vi "Set Dev Format.vi"(8 "error in (no error)":errorcluster, 9 "firmware revision":string(combo), 10 "dev format":T1 {"loss format (0)" min=0 max=4; "cap format (0)" min=0 max=4}, 11 "VISA resource name":refnum<visa-resource-name>) -> (0 "error out":errorcluster, 2 "bridge error":T2, 3 "VISA resource name out":refnum<visa-resource-name>)   [LabVIEW 2024, in "Andeen-Hagerling 2700A.lvlib"]
doc: "Set the value of the deviation mode format parameter.\n\n0 - Deviation measurement results are\n reported in absolute pF and jpF units. A\n measurement at the Deviation Setpoint will\n be reported as DPointC pF and DPointL\n jpF.\n1 - Deviation measurement results are\n reported as simple differences from the\n Deviation Setpoint in units of pF and jpF.\n A measurement at the Deviation Setpoint\n will be reported as 0 pF and 0 jpF.\n2 Deviation measurement results are\n reported as differences from the Deviation\n Setpoint as a percentage of the Deviation\n Setpoint. A measurement at the Deviation\n Setpoint will be reported as 0% for both\n capacitance and loss.\n3 Deviation measurement results are\n reported as differences from the Deviation\n Setpoint as a percentage of the deviation\n input span. Measurement values at the\n DBndLo and DBndUp bounds will be\n reported as -50% and +50% respectively.\n4 Deviation measurement results are\n reported as differences from the Deviation\n Setpoint as a percentage of the deviation\n input span. Measurement values at the\n DBndLo and DBndUp bounds will be\n reported as -100% and +100% respectively."
uses:
  Andeen-Hagerling 2700A.lvlib
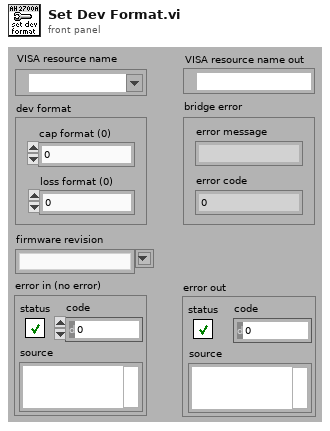
[diagram p1: front panel]
types:
  T1 = cluster{"cap format (0)":i32, "loss format (0)":i32}
  T2 = cluster{"error message":string, "error code":i32}
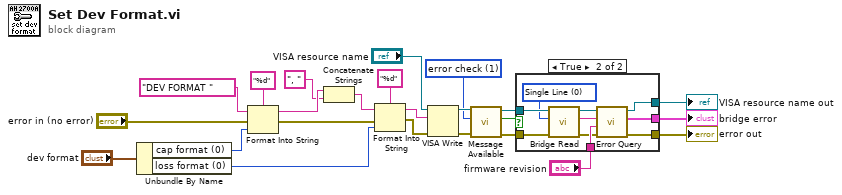
[diagram p0: block diagram]
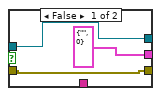
[diagram p2: hidden frame]
diagram:
  w1 = u16 1 items=["none", "error check", "multiline read", "infinite"] ("delay")
  n1 = Unbundle By Name("dev format") -> ("cap format (0)"=w3:i32, "loss format (0)"=w2:i32)
  n2 = Format Into String(format string="%d", initial string="DEV FORMAT " ("command"), error in="error in (no error)", w3) -> (resulting string=w21:string, error out=w22:errorcluster)
  n3 = Concatenate Strings(w21, ", " ("command")) -> (w15:string)
  n4 = Format Into String(format string="%d", initial string=w15, error in=w22, w2) -> (resulting string=w17:string, error out=w18:errorcluster)
  n5 = VISA Write(VISA resource name="VISA resource name", write buffer=w17, error in (no error)=w18) -> (VISA resource name out=w9:refnum<visa-resource-name>, error out=w8:errorcluster)  [unwired: 1 out]
  n6 = call "Message Available.vi"("error in (no error)"=w8, "delay"=w1, "VISA resource name"=w9) -> ("error out"=w11:errorcluster, "message available"=w13:bool, "VISA resource name out"=w12:refnum<visa-resource-name>)  [unwired: 6 in]
  n7 = case shown="True" w13 {
    tunnel: w12 -> [w26 w30]
    tunnel: w11 -> [w27 w29]
    tunnel: "firmware revision" -> [_ w37]
    tunnel: [w27 w36] -> w7
    tunnel: [w26 w35] -> w6
    tunnel: [T2 {"error message"="", "error code"=0} ("bridge error") w34] -> w5
    frame False {
    }
    frame True {
      w28 = u16 0 items=["Single Line", "Multi-Line"] ("Multiline")
      n8 = call "Bridge Read.vi"("error in (no error)"=w29, "multiline"=w28, "VISA resource name"=w30) -> ("error out"=w31:errorcluster, "read buffer"=w32:string, "VISA resource name out"=w33:refnum<visa-resource-name>)  [unwired: 6 in]
      n9 = call "Error Query.vi"("error in (no error)"=w31, "firmware revision"=w37, "measurement line"=w32, "VISA resource name"=w33) -> ("error out"=w36:errorcluster, "bridge error"=w34:T2, "VISA resource name out"=w35:refnum<visa-resource-name>)  [unwired: 5 in]
    }
  }
  "VISA resource name out" <- w6
  "error out" <- w7
  "bridge error" <- w5
